vi "Main.vi"() -> ()   [LabVIEW 2020, in "Polar Bear Plus All-in-One Plugin.lvlib"]
doc: "Main user interface for the Polar Bear Plus Flow Synthesiser controller and plugin."
uses:
  Polar Bear Plus All-in-One Plugin.lvlib
  support/Message Queue/Message Queue.lvlib
  <vilib>/Utility/error.llb/Error Cluster From Error Code.vi
  <vilib>/ErrorRing/Error Ring.xnode
  support/User Event - Stop/User Event - Stop.lvlib
  process loops/UI Manager/UI Data.ctl
  Typedefs/System Control Data.ctl
  process loops/Acquisition/Acquisition.lvlib
  process loops/Instrument Manager/Instrument Manager.lvlib
  process loops/Remote Connection Manager/Remote Connection Manager.lvlib
  process loops/Logging/Logging.lvlib
  process loops/Instrument Manager/Instrument State.ctl
  process loops/UI Manager/UI Display State.ctl
  process loops/Logging/Logging Configuration.ctl
  process loops/UI Manager/Data Display Loop Data.ctl
  <instrlib>/RxnRover/Driver Polar Bear Plus/heater_parent/heater_parent.lvclass
panel:
  in  "Ramp Rate":dbl format="%.3f °C"
  out "Heat Switch Active":bool
  in  "Time Interval (sec)":i32=1200
  out "Temperature Graph":cluster{timestamp[], dbl[]}[](graph)
  in  "Config Log Btn":bool
  in  "Sampling rate\n(sec/sample)":dbl=1.0 min=0.1 step=0.1
  in  "Log Data":bool
  in  "Stop Btn":bool=TRUE
  in  "Run Btn":bool
  out "Temperature Ind":dbl format="%.3f °C"
  in  "Setpoint":dbl format="%.3f °C"
  # "Polar Bear Plus Heater"
  # "Config"
  # "Instrument Control"
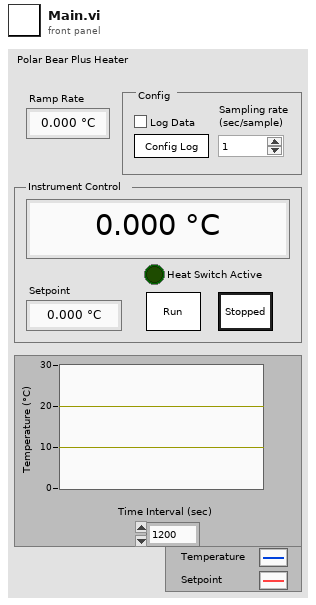
[diagram p1: front panel]
types:
  T1 = typedef "Polar Bear Plus All-in-One Plugin.lvlib/Data Display Loop Data.ctl" = cluster{"Data Timestamps":timestamp[], "Data Values":dbl[], "Setpoint":dbl[], "Previous Run State":bool}
  T2 = typedef "Polar Bear Plus All-in-One Plugin.lvlib/Instrument Manager.lvlib/Instrument State.ctl" = cluster{"Setpoint":dbl, "Running":bool, "Running Since":timestamp, "Data Point":cluster{"Time Stamp":timestamp, "Value":dbl}, "Sampling Rate (sec/sample)":dbl, "Ramp Rate":dbl, "Heat Switch Active?":bool, "Driver Object":refnum<class "heater_parent.lvclass">}
  T3 = typedef "Polar Bear Plus All-in-One Plugin.lvlib/Message Queue.lvlib/All Message Queues.ctl" = cluster{"System Control":refnum<queue>, "Instrument":refnum<queue>, "Remote":refnum<queue>, "UI":refnum<queue>, "Acquisition":refnum<queue>, "Logging":refnum<queue>}
  T4 = typedef "Polar Bear Plus All-in-One Plugin.lvlib/UI Display State.ctl" = enum16{"Shown", "Hidden"}
  T5 = enum8{"Enabled", "Disabled", "Disabled and Grayed Out"}
  T6 = typedef "Polar Bear Plus All-in-One Plugin.lvlib/UI Data.ctl" = cluster{"VISA Resource Ind":refnum<vi>, "Setpoint Ctl":refnum<vi>, "Run Btn":refnum<vi>, "Stop Btn":refnum<vi>, "Temperature Ind":refnum<vi>, "Log Data":refnum<vi>, "Config Log Btn":refnum<vi>, "Sampling rate\n(sec/sample)":refnum<vi>, "Temperature Graph":refnum<vi>}
  T7 = typedef "Polar Bear Plus All-in-One Plugin.lvlib/Logging.lvlib/Logging Configuration.ctl" = cluster{"Log Directory Path":path, "Log File Path":path, "Log File Prefix":string, "Log File Extension":string, "File Delimiter":string, "Header Info":string[][], "Channels":string[], "Log Instrument Runs":bool}
  T8 = typedef "Polar Bear Plus All-in-One Plugin.lvlib/System Control Data.ctl" = cluster{"Example Value <Replace Me>":dbl, "Log Runs":bool, "Clone":bool}
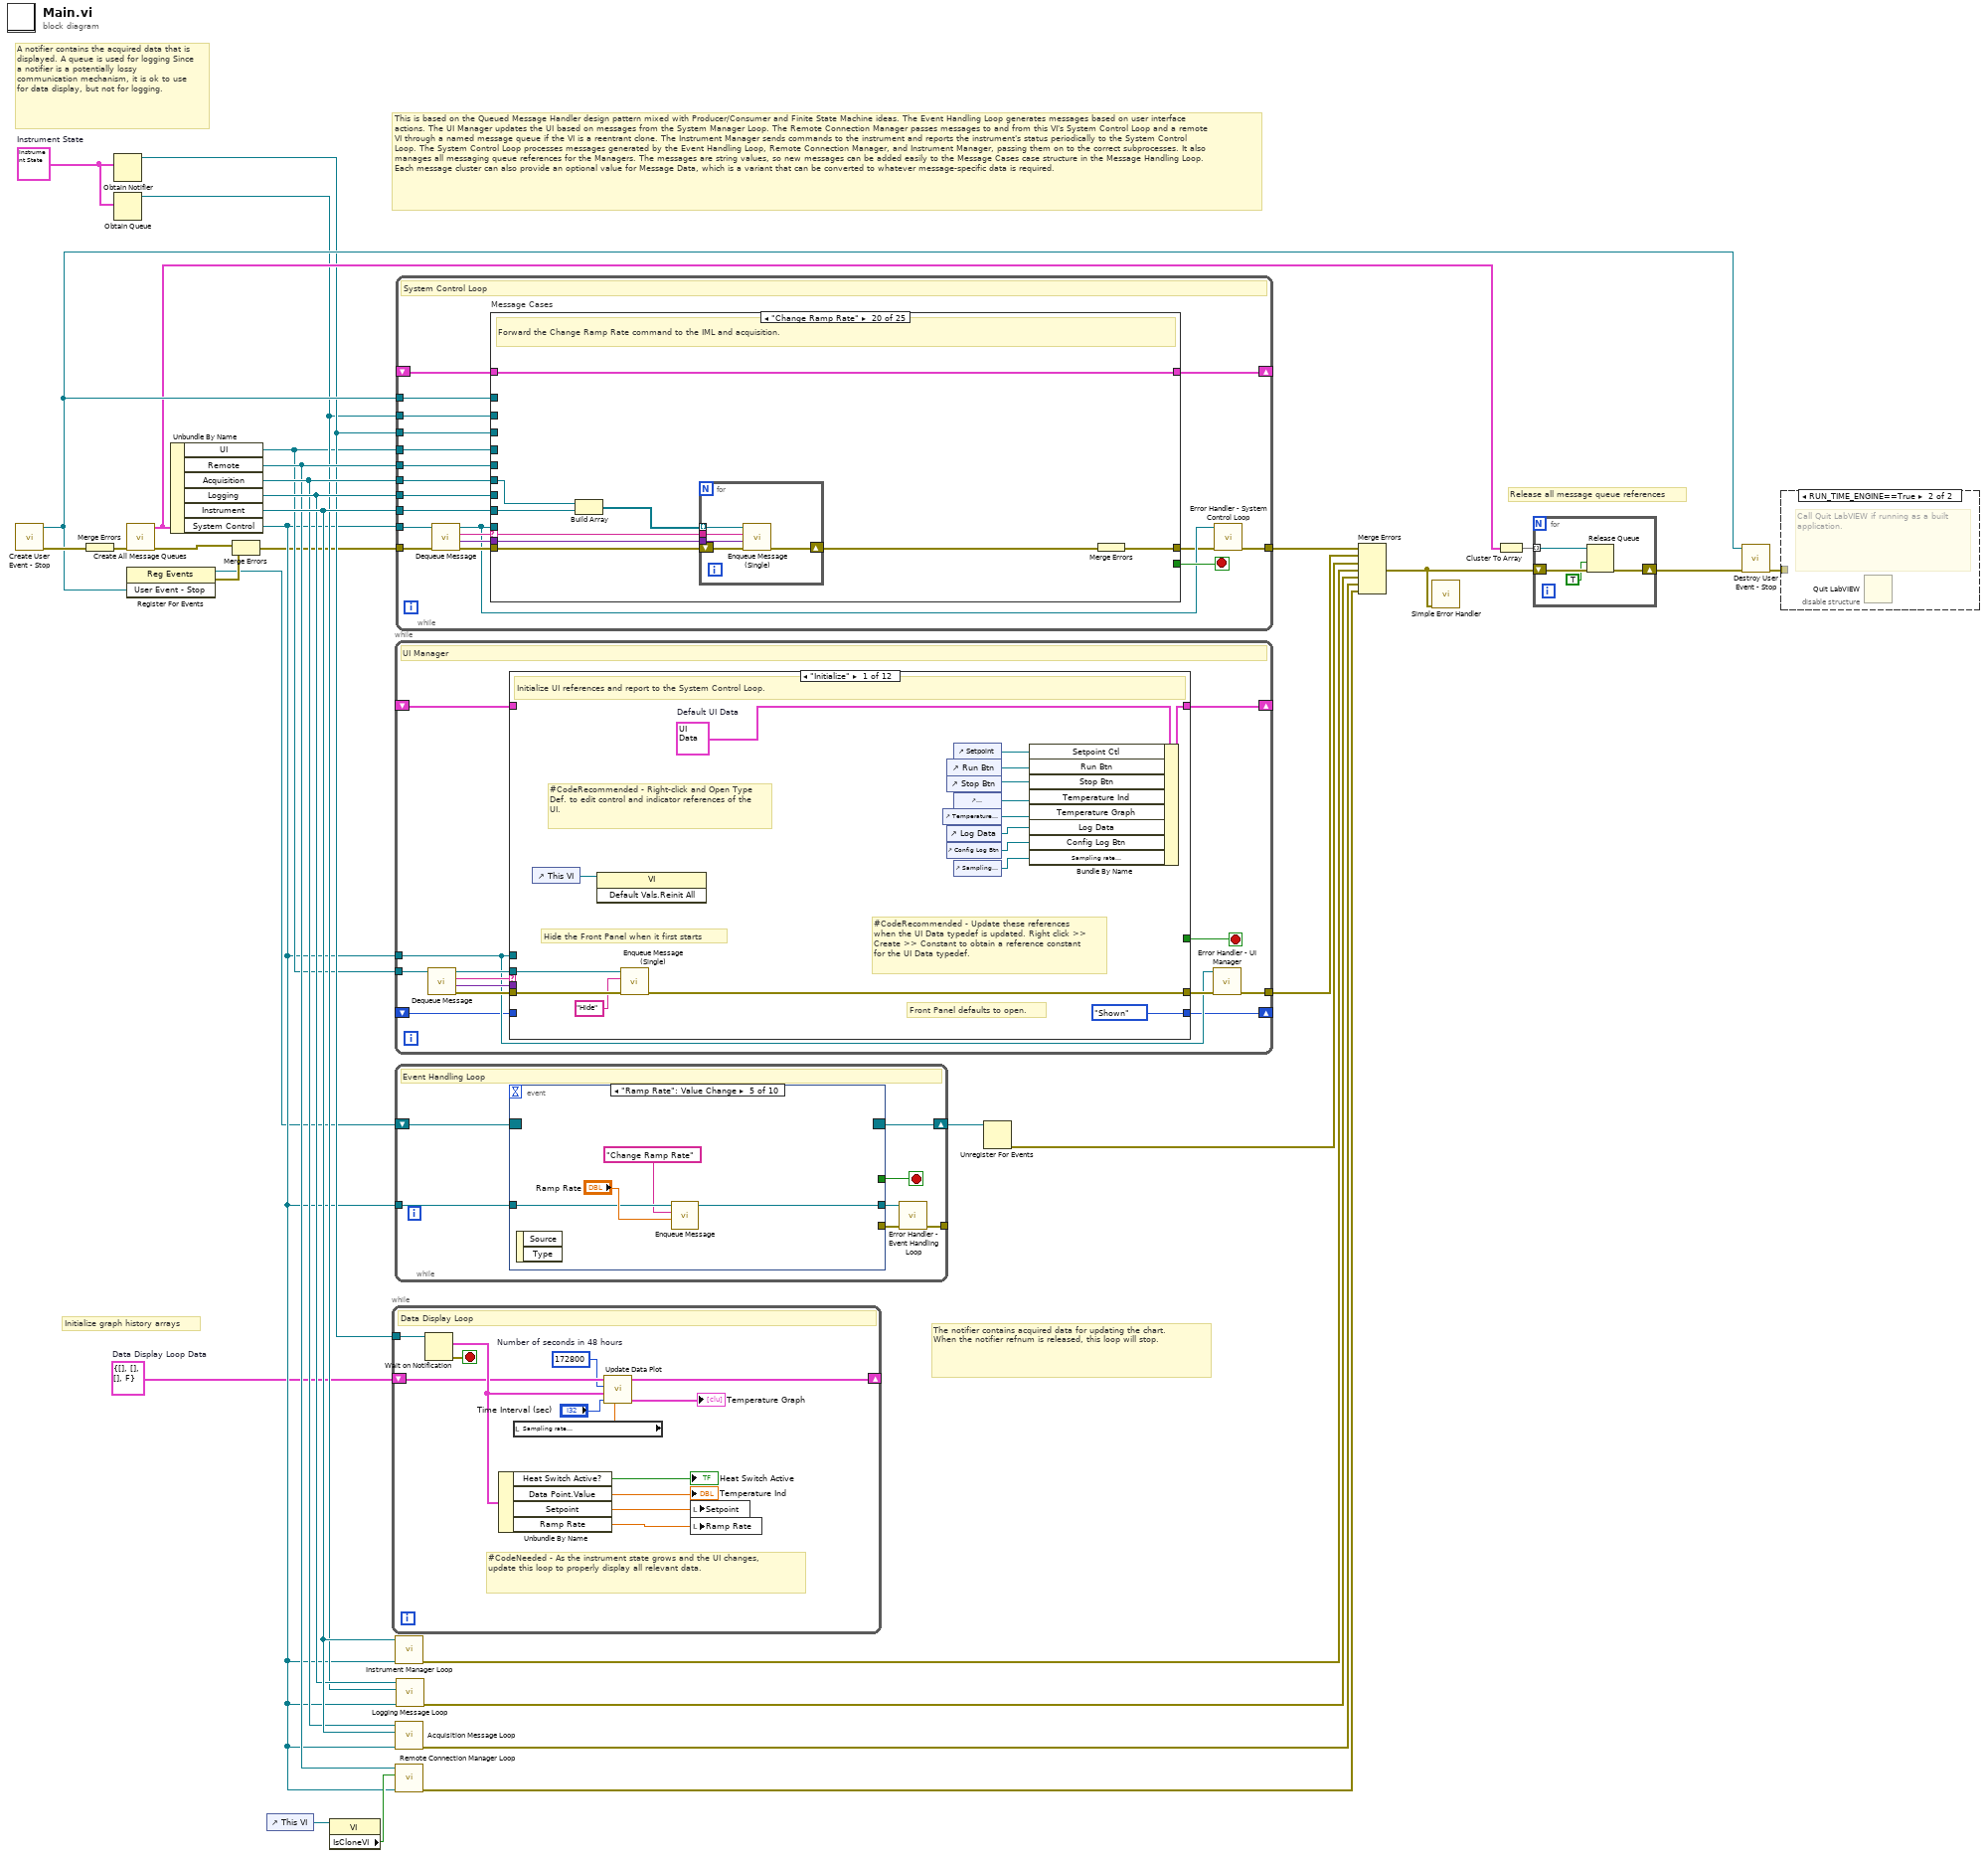
[diagram p0: block diagram]
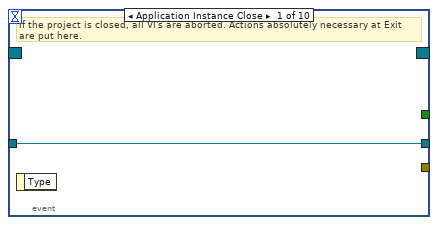
[diagram p2: hidden frame]
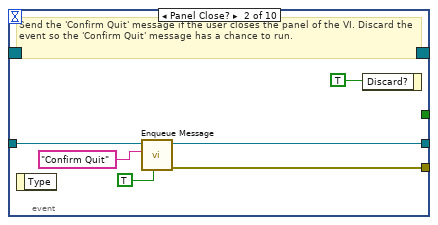
[diagram p3: hidden frame]
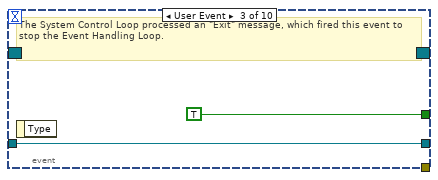
[diagram p4: hidden frame]
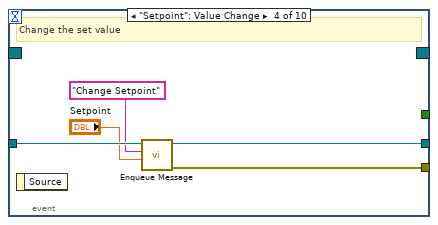
[diagram p5: hidden frame]
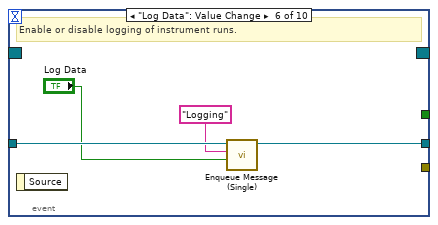
[diagram p6: hidden frame]
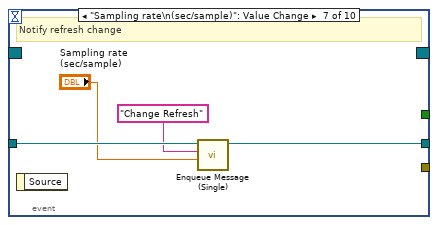
[diagram p7: hidden frame]
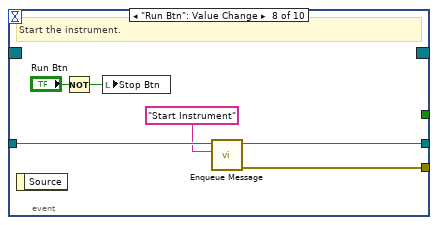
[diagram p8: hidden frame]
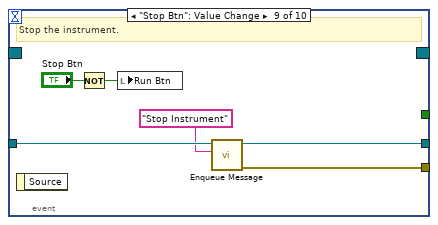
[diagram p9: hidden frame]
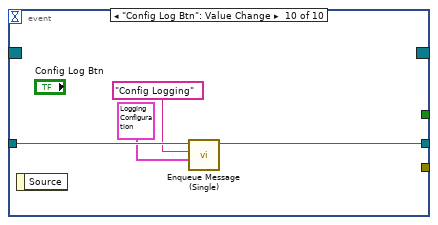
[diagram p10: hidden frame]
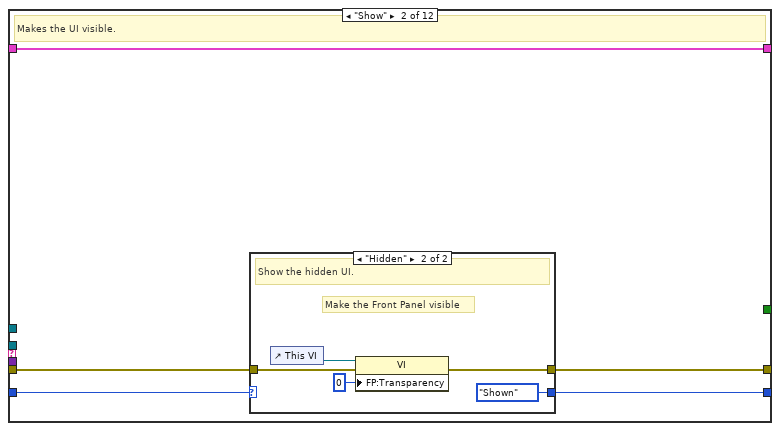
[diagram p11: hidden frame]
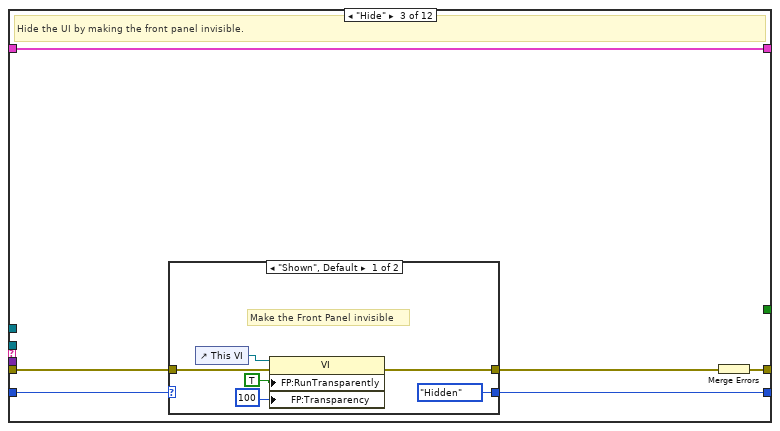
[diagram p13: hidden frame]
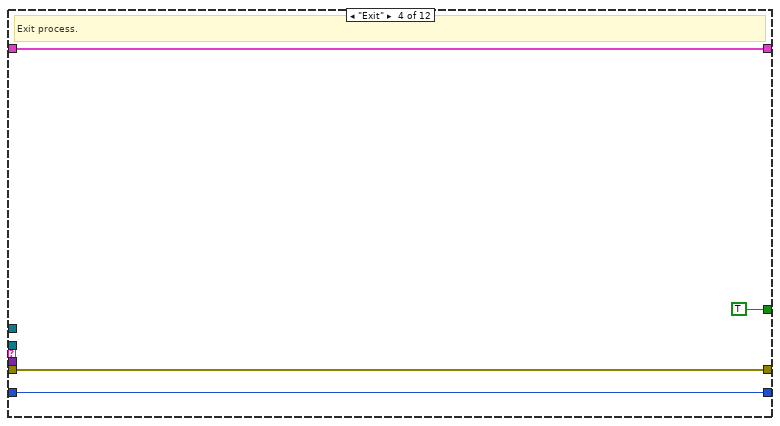
[diagram p15: hidden frame]
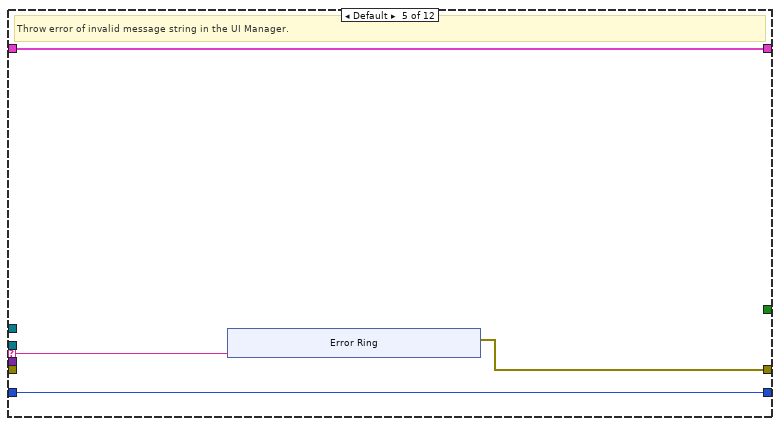
[diagram p16: hidden frame]
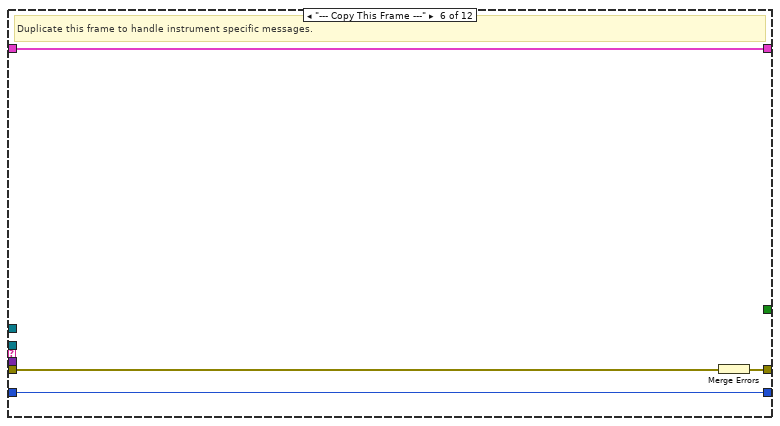
[diagram p17: hidden frame]
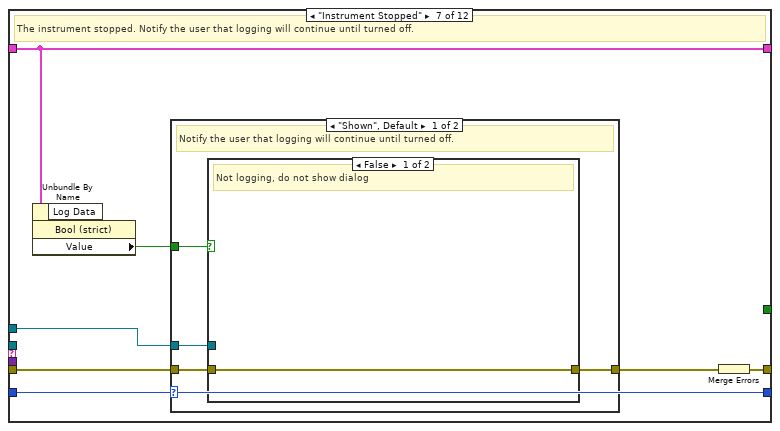
[diagram p18: hidden frame]
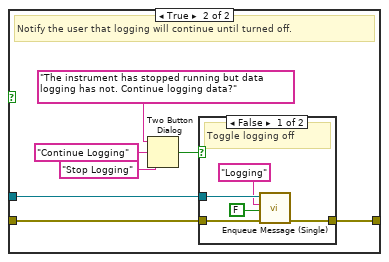
[diagram p19: hidden frame]
diagram:
  w1 = T1 {"Data Timestamps"=[], "Data Values"=[], "Setpoint"=[], "Previous Run State"=FALSE}  # Data Display Loop Data
  w7 = T2 {"Setpoint"=0.0, "Running"=FALSE, "Running Since"=timestamp(0 s since 1904-01-01), "Data Point"={"Time Stamp"=timestamp(0 s since 1904-01-01), "Value"=0.0}, "Sampling Rate (sec/sample)"=0.0, "Ramp Rate"=0.0, "Heat Switch Active?"=FALSE, "Driver Object"=refnum}  # Instrument State
  # "Initialize graph history arrays"
  # "A notifier contains the acquired data that is displayed. A queue is used for logging Since a notifier is a potentially lossy communication mechanism, it is ok to use for data display, but not for logging."
  # "The notifier contains acquired data for updating the chart. When the notifier refnum is released, this loop will stop."
  # "Release all message queue references"
  # "This is based on the Queued Message Handler design pattern mixed with Producer/Consumer and Finite State Machine ideas. The Event Handling Loop generates messages based on user interface actions. The UI Manager updates the UI based on messages from the System Manager Loop. The Remote Connection Manager passes messages to and from this VI's System Control Loop and a remote VI through a named message queue if the VI is a reentrant clone. The Instrument Manager sends commands to the instrument and reports the instrument's status periodically to the System Control Loop. The System Control Loop processes messages generated by the Event Handling Loop, Remote Connection Manager, and Instrument Manager, passing them on to the correct subprocesses. It also manages all messaging queue references for the Managers. The messages are string values, so new messages can be added easily to the Message Cases case structure in the Message Handling Loop.  Each message cluster can also provide an optional value for Message Data, which is a variant that can be converted to whatever message-specific data is required."
  n1 = call "Create User Event - Stop.vi"() -> ("error out"=w26:errorcluster, "User Event - Stop"=w22:refnum<user-event>)  [unwired: 10 in]
  n2 = Merge Errors(w26) -> (w25:errorcluster)
  n3 = Obtain Notifier(notification data type=w7) -> (notifier out=w8:refnum<notifier>)  [unwired: 3 in, 2 out]
  n4 = Obtain Queue(element data type=w7) -> (queue out=w6:refnum<queue>)  [unwired: 4 in, 2 out]
  n5 = call "Create All Message Queues.vi"("error in (no error)"=w25) -> ("error out"=w28:errorcluster, "Message Queues out"=w11:T3)  [unwired: 9 in]
  n6 = register-events(w22) -> (reference out=w2:refnum<event-registration>, error out=w13:errorcluster)  [unwired: 2 in]
  n7 = Unbundle By Name(w11) -> ("UI"=w5:refnum<queue>, "Remote"=w29:refnum<queue>, "Acquisition"=w30:refnum<queue>, "Logging"=w31:refnum<queue>, "Instrument"=w32:refnum<queue>, "System Control"=w4:refnum<queue>)
  n8 = Merge Errors(w28, w13) -> (w3:errorcluster)
  n9 = control-ref of="This VI"() -> (w21:refnum<vi>)
  n10 = property class="VI"(reference=w21) -> ("IsCloneVI"=w20:bool)  [unwired: 1 in, 2 out]
  n11 = while "Data Display Loop" {
    tunnel: w8 -> [w45]
    shift-right: [w38] -> _
    shift-left: w1 -> [w39]
    stop <- w44 stop-if-true
    w35 = 172800  # Number of seconds in 48 hours
    # "#CodeNeeded - As the instrument state grows and the UI changes, update this loop to properly display all relevant data."
    # "Data Display Loop"
    n12 = Wait on Notification(notifier=w45) -> (notification=w40:T2, error out=w44:errorcluster)  [unwired: 3 in, 2 out]
    n13 = Unbundle By Name(w40) -> ("Heat Switch Active?"=→"Heat Switch Active":bool, "Data Point.Value"=→"Temperature Ind":dbl, "Setpoint"=w42:dbl, "Ramp Rate"=w33:dbl)
    n14 = local read "Sampling rate\n(sec/sample)"() -> (w36:dbl)
    n15 = call "Update Data Plot.vi"("Sample Rate (sec/sample)"=w36, "Time interval (s)"="Time Interval (sec)", "Instrument State"=w40, "History length"=w35, "Graph History Arrays in"=w39) -> ("Updated Plot History"=→"Temperature Graph":cluster{timestamp[], dbl[]}[], "Graph History Arrays out"=w38:T1)  [unwired: 5 in]
    n16 = local write "Setpoint"(w42) -> ()
    n17 = local write "Ramp Rate"(w33) -> ()
  }
  n18 = while {
    tunnel: w5 -> [w58]
    tunnel: w4 -> [w49]
    tunnel: [w50] -> w19
    shift-right: [w53] -> _
    shift-left: _ -> [w52]
    shift-right: [w47] -> _
    shift-left: _ -> [w46]
    stop <- w48 stop-if-true
    # "UI Manager"
    n19 = call "Dequeue Message.vi"("Message Queue"=w58) -> ("error out"=w56:errorcluster, "Message Data"=w54:variant, "Message"=w55:string, "dup Message Queue"=w57:refnum<queue>)  [unwired: 7 in]
    n20 = case shown="\"Initialize\"" w55 {
      selector: w55 -> [_ _ _ _ w108 _ _ _ _ _ _ _]
      tunnel: w57 -> [w66 _ _ _ _ _ _ _ _ _ _ _]
      tunnel: w56 -> [w71 w78 w90 w104 _ w117 w125 w153 w161 w169 w180 w191]
      tunnel: w54 -> [_ _ _ _ _ _ _ _ _ w168 w178 w189]
      tunnel: w49 -> [_ _ _ _ _ _ w123 _ _ _ _ _]
      tunnel: [w67 w77 w91 w104 w107 w118 w127 w154 w162 w170 w181 w192] -> w51
      tunnel: [w73 w79 w92 w103 w106 w119 w122 w149 w155 w164 w172 w183] -> w53
      tunnel: w52 -> [_ w79 w92 w103 w106 w119 w122 w149 w155 w164 w172 w183]
      tunnel: [_ _ _ TRUE _ _ _ _ _ _ _ _] -> w48
      tunnel: w46 -> [_ w76 w88 w101 w105 w116 w126 w152 w160 w166 w173 w184]
      tunnel: [UI_Display_State."Shown" ("UI Display State") w75 w87 w101 w105 w116 w126 w152 w160 w166 w173 w184] -> w47
      frame "Initialize" {
        w74 = T6 {"VISA Resource Ind"=refnum, "Setpoint Ctl"=refnum, "Run Btn"=refnum, "Stop Btn"=refnum, "Temperature Ind"=refnum, "Log Data"=refnum, "Config Log Btn"=refnum, "Sampling rate\n(sec/sample)"=refnum, "Temperature Graph"=refnum}  # Default UI Data
        # "Front Panel defaults to open."
        # "Hide the Front Panel when it first starts"
        # "#CodeRecommended - Update these references when the UI Data typedef is updated. Right click >> Create >> Constant to obtain a reference constant for the UI Data typedef."
        # "#CodeRecommended - Right-click and Open Type Def. to edit control and indicator references of the UI."
        # "Initialize UI references and report to the System Control Loop."
        n21 = control-ref of="This VI"() -> (w59:refnum<vi>)
        n22 = invoke class="VI" method="Default Vals.Reinit All"(reference=w59) -> ()  [unwired: 2 in, 3 out]
        n23 = call "Enqueue Message (Single).vi"("error in (no error)"=w71, "Message"="Hide", "Message Queue"=w66) -> ("error out"=w67:errorcluster)  [unwired: 7 in, 1 out]
        n24 = control-ref of="Temperature Graph"() -> (w63:refnum<vi>)
        n25 = control-ref of="Run Btn"() -> (w69:refnum<vi>)
        n26 = control-ref of="Stop Btn"() -> (w70:refnum<vi>)
        n27 = control-ref of="Log Data"() -> (w62:refnum<vi>)
        n28 = control-ref of="Config Log Btn"() -> (w61:refnum<vi>)
        n29 = control-ref of="Setpoint"() -> (w72:refnum<vi>)
        n30 = control-ref of="Temperature Ind"() -> (w68:refnum<vi>)
        n31 = control-ref of="Sampling rate (sec/sample)"() -> (w60:refnum<vi>)
        n32 = Bundle By Name(cluster=w74, "Setpoint Ctl"=w72, "Run Btn"=w69, "Stop Btn"=w70, "Temperature Ind"=w68, "Temperature Graph"=w63, "Log Data"=w62, "Config Log Btn"=w61, "Sampling rate\n(sec/sample)"=w60) -> (w73:T6)
      }
      frame "Show" {
        # "Makes the UI visible."
        n33 = case shown="\"Hidden\"" w76 {
          selector: w76 -> [w81 _]
          tunnel: w78 -> [w80 w86]
          tunnel: [w80 w84] -> w77
          tunnel: [w81 UI_Display_State."Shown" ("UI Display State")] -> w75
          frame "Shown", Default {
            # "Do nothing if UI is already shown."
          }
          frame "Hidden" {
            # "Make the Front Panel visible"
            # "Show the hidden UI."
            n34 = control-ref of="This VI"() -> (w85:refnum<vi>)
            n35 = property class="VI"(reference=w85, error in=w86, "FP:Transparency"=u8 0 ("Front Panel Window:Transparency")) -> (error out=w84:errorcluster)  [unwired: 1 out]
          }
        }
      }
      frame "Hide" {
        # "Hide the UI by making the front panel invisible."
        n36 = case shown="\"Shown\", Default" w88 {
          selector: w88 -> [_ w100]
          tunnel: w90 -> [w95 w99]
          tunnel: [w94 w99] -> w89
          tunnel: [UI_Display_State."Hidden" ("UI Display State") w100] -> w87
          frame "Shown", Default {
            # "Make the Front Panel invisible"
            n37 = control-ref of="This VI"() -> (w98:refnum<vi>)
            n38 = property class="VI"(reference=w98, error in=w95, "FP:RunTransparently"=TRUE ("Front Panel Window:Run VI Transparently"), "FP:Transparency"=u8 100 ("Front Panel Window:Transparency")) -> (error out=w94:errorcluster)  [unwired: 1 out]
          }
          frame "Hidden" {
          }
        }
        n39 = Merge Errors(w89) -> (w91:errorcluster)
      }
      frame "Exit" {
        # "Exit process."
      }
      frame Default {
        # "Throw error of invalid message string in the UI Manager."
        n40 = xnode "Error Ring"("parameter 0"=w108) -> ("error out"=w107:errorcluster)
      }
      frame "--- Copy This Frame ---" {
        # "Duplicate this frame to handle instrument specific messages."
        n41 = Merge Errors(w117) -> (w118:errorcluster)
      }
      frame "Instrument Stopped" {
        # "The instrument stopped. Notify the user that logging will continue until turned off."
        n42 = Unbundle By Name(w122) -> ("Log Data"=w121:refnum<vi>)
        n43 = property class="Bool (strict)"(reference=w121) -> ("Value"=w120:bool)  [unwired: 1 in, 2 out]
        n44 = case shown="\"Shown\", Default" w126 {
          tunnel: w125 -> [w131 w146]
          tunnel: [w130 w146] -> w124
          tunnel: w123 -> [w129 _]
          tunnel: w120 -> [w128 _]
          frame "Shown", Default {
            # "Notify the user that logging will continue until turned off."
            n45 = case shown="False" w128 {
              tunnel: w131 -> [w132 w135]
              tunnel: [w132 w134] -> w130
              tunnel: w129 -> [_ w133]
              frame False {
                # "Not logging, do not show dialog"
              }
              frame True {
                # "Notify the user that logging will continue until turned off."
                n46 = Two Button Dialog(message="The instrument has stopped running but data logging has not. Continue logging data?", 1:"Stop Logging" ("F button name (\"Cancel\")"), 2:"Continue Logging" ("T button name (\"OK\")")) -> (T button?=w136:bool)
                n47 = case shown="False" w136 {
                  tunnel: w135 -> [w144 w145]
                  tunnel: [w143 w145] -> w134
                  tunnel: w133 -> [w142 _]
                  frame False {
                    # "Toggle logging off"
                    n48 = call "Enqueue Message (Single).vi"("error in (no error)"=w144, "Message Data"=FALSE, "Message"="Logging", "Message Queue"=w142) -> ("error out"=w143:errorcluster)  [unwired: 6 in, 1 out]
                  }
                  frame True {
                    # "Continues logging. Do nothing more"
                  }
                }
              }
            }
          }
          frame "Hidden" {
            # "Hidden, do not show dialog"
          }
        }
        n49 = Merge Errors(w124) -> (w127:errorcluster)
      }
      frame "Logging Started" {
        # "Indicate that logging started."
        n50 = Unbundle By Name(w149) -> ("Log Data"=w151:refnum<vi>)
        n51 = property class="Bool (strict)"(reference=w151, "Value"=TRUE ("Log Data")) -> ()  [unwired: 1 in, 2 out]
        n52 = Unbundle By Name(w149) -> ("Config Log Btn"=w148:refnum<vi>)
        n53 = property class="Bool"(reference=w148, "DisabledEnum"=T5."Disabled and Grayed Out" ("Disabled")) -> ()  [unwired: 1 in, 2 out]
        n54 = Merge Errors(w153) -> (w154:errorcluster)
      }
      frame "Logging Stopped" {
        # "Indicate that logging stopped."
        n55 = Unbundle By Name(w155) -> ("Log Data"=w159:refnum<vi>)
        n56 = property class="Bool (strict)"(reference=w159, "Value"=FALSE ("Log Data")) -> ()  [unwired: 1 in, 2 out]
        n57 = Unbundle By Name(w155) -> ("Config Log Btn"=w157:refnum<vi>)
        n58 = property class="Bool"(reference=w157, "DisabledEnum"=T5."Enabled" ("Disabled")) -> ()  [unwired: 1 in, 2 out]
        n59 = Merge Errors(w161) -> (w162:errorcluster)
      }
      frame "Change Refresh" {
        # "Update sample rate multiplier in the UI data chart and config indicator."
        n60 = Unbundle By Name(w164) -> ("Sampling rate\n(sec/sample)"=w165:refnum<vi>)
        n61 = Variant To Data(type=0.0, Variant=w168) -> (data=w163:dbl)  [unwired: 1 in, 1 out]
        n62 = property class="DigNum (strict)"(reference=w165, "Value"=w163) -> ()  [unwired: 1 in, 2 out]
        n63 = Merge Errors(w169) -> (w170:errorcluster)
      }
      frame "Display Units - Temperature Ind" {
        # "#CodeRecommended - If this format string is changed, update it on the front panel indicator as well."
        # "Change the units of the display."
        n64 = Variant To Data(type="", Variant=w178) -> (data=w176:string)  [unwired: 1 in, 1 out]
        n65 = call <vilib>:"Space Constant.vi"() -> ("String"=w177:string)
        n66 = Concatenate Strings("%.3f" ("string"), w177, w176) -> (w174:string)
        n67 = Unbundle By Name(w172) -> ("Temperature Ind"=w171:refnum<vi>)
        n68 = property on="Property Node" class="DigNum (strict)"(reference=w171, "FormatString"=w174) -> ()  [unwired: 1 in, 2 out]
        n69 = Merge Errors(w180) -> (w181:errorcluster)
      }
      frame "Display Units - Setpoint" {
        # "#CodeRecommended - If this format string is changed, update it on the front panel indicator as well."
        # "Change the units of the setpoint display."
        n70 = Variant To Data(type="", Variant=w189) -> (data=w187:string)  [unwired: 1 in, 1 out]
        n71 = call <vilib>:"Space Constant.vi"() -> ("String"=w188:string)
        n72 = Concatenate Strings("%.3f" ("string"), w188, w187) -> (w185:string)
        n73 = Unbundle By Name(w183) -> ("Setpoint Ctl"=w182:refnum<vi>)
        n74 = property on="Property Node" class="DigNum (strict)"(reference=w182, "FormatString"=w185) -> ()  [unwired: 1 in, 2 out]
        n75 = Merge Errors(w191) -> (w192:errorcluster)
      }
    }
    n76 = call "Error Handler - UI Manager.vi"("error in (no error)"=w51, "Message Queue"=w49) -> ("dup error in"=w50:errorcluster)  [unwired: 8 in, 1 out]
  }
  n77 = while {
    tunnel: w4 -> [w199]
    shift-right: [w197] -> w23
    shift-left: w2 -> [w198]
    tunnel: [w193] -> _
    stop <- w195 stop-if-true
    # "Event Handling Loop"
    n78 = event shown="[4] \"Ramp Rate\": Value Change" {
      selector: w198 -> [_ _ _ _ _ _ _ _ _ _]
      dyn-events: [_ _ _ _ _ _ _ _ _ _] -> w197
      timeout: _ -> [_ _ _ _ _ _ _ _ _ _]
      tunnel: [_ _ TRUE ("Discard?") _ _ _ _ _ _ _] -> w195
      tunnel: w199 -> [w200 w205 w208 w213 w216 w221 w225 w231 w237 w241]
      tunnel: [_ w204 _ w210 _ _ _ w229 w235 _] -> w196
      tunnel: [w200 w203 w208 w212 w215 w220 w224 w230 w236 w240] -> w194
      event Application Instance Close {
        # "If the project is closed, all VI's are aborted. Actions absolutely necessary at Exit are put here."
        n79 = event-data() -> ()  [unwired: 1 in, 1 out]
      }
      event Panel Close? {
        # "Send the 'Confirm Quit' message if the user closes the panel of the VI. Discard the event so the 'Confirm Quit' message has a chance to run."
        n80 = event-data() -> ()  [unwired: 1 in, 1 out]
        n81 = call-poly "Enqueue Message.vi"("Priority Message? (F)"=TRUE, "Message"="Confirm Quit", "Message Queue"=w205) -> ("error out"=w204:errorcluster, "dup Message Queue"=w203:refnum<queue>)  [unwired: 7 in]
        n82 = event-data("Discard?"=TRUE) -> ()  [unwired: 1 in, 1 out]
      }
      event User Event {
        # "The System Control Loop processed an \"Exit\" message, which fired this event to stop the Event Handling Loop."
        n83 = event-data() -> ()  [unwired: 1 in, 1 out]
      }
      event "Setpoint": Value Change {
        # "Change the set value"
        n84 = event-data() -> ()  [unwired: 1 in, 1 out]
        n85 = call-poly "Enqueue Message.vi"("Message Data"="Setpoint", "Message"="Change Setpoint", "Message Queue"=w213) -> ("error out"=w210:errorcluster, "dup Message Queue"=w212:refnum<queue>)  [unwired: 7 in]
      }
      event "Ramp Rate": Value Change {
        n86 = event-data() -> ()  [unwired: 1 in, 2 out]
        n87 = call-poly "Enqueue Message.vi"("Message Data"="Ramp Rate", "Message"="Change Ramp Rate", "Message Queue"=w216) -> ("dup Message Queue"=w215:refnum<queue>)  [unwired: 7 in, 1 out]
      }
      event "Log Data": Value Change {
        # "Enable or disable logging of instrument runs."
        n88 = event-data() -> ()  [unwired: 1 in, 1 out]
        n89 = call "Enqueue Message (Single).vi"("Message Data"="Log Data", "Message"="Logging", "Message Queue"=w221) -> ("dup Message Queue"=w220:refnum<queue>)  [unwired: 7 in, 1 out]
      }
      event "Sampling rate\n(sec/sample)": Value Change {
        # "Notify refresh change"
        n90 = event-data() -> ()  [unwired: 1 in, 1 out]
        n91 = call "Enqueue Message (Single).vi"("Message Data"="Sampling rate\n(sec/sample)", "Message"="Change Refresh", "Message Queue"=w225) -> ("dup Message Queue"=w224:refnum<queue>)  [unwired: 7 in, 1 out]
      }
      event "Run Btn": Value Change {
        # "Start the instrument."
        n92 = event-data() -> ()  [unwired: 1 in, 1 out]
        n93 = Not(x="Run Btn") -> (.not. x?=w226:bool)
        n94 = local write "Stop Btn"(w226) -> ()
        n95 = call-poly "Enqueue Message.vi"("Message"="Start Instrument", "Message Queue"=w231) -> ("error out"=w229:errorcluster, "dup Message Queue"=w230:refnum<queue>)  [unwired: 8 in]
      }
      event "Stop Btn": Value Change {
        # "Stop the instrument."
        n96 = event-data() -> ()  [unwired: 1 in, 1 out]
        n97 = Not(x="Stop Btn") -> (.not. x?=w232:bool)
        n98 = local write "Run Btn"(w232) -> ()
        n99 = call-poly "Enqueue Message.vi"("Message"="Stop Instrument", "Message Queue"=w237) -> ("error out"=w235:errorcluster, "dup Message Queue"=w236:refnum<queue>)  [unwired: 8 in]
      }
      event "Config Log Btn": Value Change {
        n100 = event-data() -> ()  [unwired: 1 in, 1 out]
        n101 = call "Enqueue Message (Single).vi"("Message Data"=T7 {"Log Directory Path"=path "", "Log File Path"=path "", "Log File Prefix"="Experiment", "Log File Extension"="csv", "File Delimiter"=",", "Header Info"=[], "Channels"=[], "Log Instrument Runs"=FALSE} ("Logging Configuration"), "Message"="Config Logging", "Message Queue"=w241) -> ("dup Message Queue"=w240:refnum<queue>)  [unwired: 7 in, 1 out]
      }
    }
    n102 = call "Error Handler - Event Handling Loop.vi"("error in (no error)"=w196, "Message Queue"=w194) -> ("dup error in"=w193:errorcluster)  [unwired: 8 in, 1 out]
  }
  n103 = call "Instrument Manager Loop.vi"("System Control"=w4, "Instrument Manager"=w32) -> ("error out"=w17:errorcluster)  [unwired: 9 in]
  n104 = call "Acquisition Message Loop.vi"("System Control"=w4, "Instrument Manager"=w32, "Acquisition"=w30) -> ("error out"=w15:errorcluster)  [unwired: 8 in]
  n105 = call "Remote Connection Manager Loop.vi"("System Control"=w4, "IsCloneVI (false)"=w20, "RCM Queue"=w29) -> ("error out"=w14:errorcluster)  [unwired: 8 in]
  n106 = while {
    tunnel: w4 -> [w252]
    shift-right: [w259] -> _
    shift-left: _ -> [w260]
    tunnel: w22 -> [w257]
    tunnel: w3 -> [w256]
    tunnel: [w250] -> w27
    tunnel: w32 -> [w248]
    tunnel: w29 -> [w247]
    tunnel: w5 -> [w246]
    tunnel: w30 -> [w245]
    tunnel: w31 -> [w244]
    tunnel: w8 -> [w243]
    tunnel: w6 -> [w242]
    stop <- w258 stop-if-true
    # "System Control Loop"
    n107 = call "Dequeue Message.vi"("error in (no error)"=w256, "Message Queue"=w252) -> ("error out"=w255:errorcluster, "Message Data"=w253:variant, "Message"=w254:string, "dup Message Queue"=w251:refnum<queue>)  [unwired: 6 in]
    n108 = case "Message Cases" shown="\"Change Ramp Rate\"" w254 {
      selector: w254 -> [_ _ _ w302 w315 w326 w344 w358 w364 _ w410 w417 w424 w431 w438 w448 w462 w477 w491 w505 w516 w523 w533 w548 w570]
      tunnel: w251 -> [_ _ w282 _ _ _ _ _ _ _ _ _ _ _ _ _ _ _ _ _ _ _ _ _ _]
      tunnel: w255 -> [w264 w279 w286 _ _ w329 w347 w362 w380 w393 w414 w421 w428 w435 w442 w451 w465 w481 w495 w509 w519 w526 _ _ _]
      tunnel: [w263 w273 w284 w305 w316 w335 w349 w363 w371 w398 w415 w422 w429 w436 w443 w452 w466 w479 w493 w507 w520 w527 w532 w547 w569] -> w249
      tunnel: w260 -> [_ w278 w285 w301 w317 w336 w350 w361 w370 w399 w416 w423 w430 w437 w444 w453 w467 w480 w494 w508 w521 w528 w531 w544 w567]
      tunnel: [w265 w278 w285 w301 w317 w336 w350 w361 w370 w397 w416 w423 w430 w437 w444 w453 w467 w480 w494 w508 w521 w528 w531 w544 w567] -> w259
      tunnel: [_ _ _ TRUE _ _ _ _ _ _ _ _ _ _ _ _ _ _ _ _ _ _ _ _ _] -> w258
      tunnel: w253 -> [_ w277 _ w306 _ w325 w343 w357 w365 w395 w411 w418 w425 w432 w439 w449 w463 w476 w490 w504 w517 w524 w534 w549 w565]
      tunnel: w257 -> [_ _ _ w303 _ _ _ _ _ _ _ _ _ _ _ _ _ _ _ _ _ _ _ _ _]
      tunnel: w248 -> [w262 _ _ w298 _ w330 _ w359 _ _ _ _ _ _ _ _ _ _ w489 w503 w515 w522 _ _ _]
      tunnel: w247 -> [_ _ _ w297 _ w333 w348 _ w375 _ _ _ _ _ _ w447 w461 _ _ _ _ _ w535 w545 w568]
      tunnel: w246 -> [_ _ _ w296 _ w332 _ _ w374 _ _ _ _ _ _ w446 w460 w474 _ _ _ _ _ w543 _]
      tunnel: w245 -> [_ _ _ w300 _ w334 _ _ w377 _ _ _ _ _ _ _ _ w475 w488 w502 _ _ w530 _ _]
      tunnel: w244 -> [_ _ _ w299 _ w331 _ _ w367 w391 w412 w419 w426 w433 w440 _ _ _ _ _ _ _ w529 _ _]
      tunnel: w243 -> [_ _ _ w293 _ _ _ _ _ _ _ _ _ _ _ _ _ _ _ _ _ _ _ _ w566]
      tunnel: w242 -> [_ _ _ w291 _ _ _ _ _ _ _ _ _ _ _ _ _ _ _ _ _ _ _ _ w562]
      frame "Initialize" {
        w266 = T8 {"Example Value <Replace Me>"=0.0, "Log Runs"=FALSE, "Clone"=FALSE}  # Default Data
        # "Initialize the system control loop and system."
        n109 = control-ref of="This VI"() -> ()  [unwired: 1 out]
        n110 = property on="Property Node" class="VI"() -> ("IsCloneVI"=w261:bool)  [unwired: 2 in, 2 out]
        n111 = Bundle By Name(cluster=w266, "Clone"=w261) -> (w265:T8)
        n112 = case shown="False" w261 {
          tunnel: w264 -> [w269 w272]
          tunnel: [w268 w272] -> w263
          tunnel: w262 -> [w267 _]
          frame False {
            # "Initiate the VISA Resource selection window if this is not a"
            n113 = call "Enqueue Message (Single).vi"("error in (no error)"=w269, "Message Data"=refnum<visa-resource-name> refnum ("VISA resource out"), "Message"="Set VISA Resource", "Message Queue"=w267) -> ("error out"=w268:errorcluster)  [unwired: 6 in, 1 out]
          }
          frame True {
            # "Reentrant clone. It is the responsibility of the RCM to send the Set VISA Resource command."
          }
        }
      }
      frame "Error" {
        # "#CodeRecommended - If you ever change the name of this \"Error\" message, you'll need to update the name in the Check Loop Error.vi as well."
        # "#CodeRecommended - Consider creating a system for logging errors in some way. These errors are for notification purposes only. Handling of specific errors should be performed in the message frames that generated the error."
        # "Error - Display an error dialog. This message is sent by the \"Error Handler\" VIs at the end of other loops in this application."
        n114 = Variant To Data(error in=w279, type=errorcluster {"status"=FALSE, "code"=0, "source"=""} ("error constant"), Variant=w277) -> (data=w275:errorcluster, error out=w274:errorcluster)
        n115 = call <vilib>:"Simple Error Handler.vi"("error in (no error)"=w275) -> ()  [unwired: 4 in, 5 out]
        n116 = Merge Errors(w274) -> (w273:errorcluster)
      }
      frame "Confirm Quit" {
        # "#CodeNeeded - If you want to provide an \"Are you sure\" dialog (or some other notification) before the application exits, place that code here. This message is typically sent from a Panel Close? event."
        # "Confirm Quit - Message that can confirm whether or not the user wants to exit the application."
        n117 = call-poly "Enqueue Message.vi"("Priority Message? (F)"=TRUE, "error in (no error)"=w286, "Message"="Exit", "Message Queue"=w282) -> ("error out"=w283:errorcluster)  [unwired: 6 in, 1 out]
        n118 = Merge Errors(w283) -> (w284:errorcluster)
      }
      frame "Exit" {
        # "Order other processes to exit"
        # "Begin the application closing procedure by sending \"Exit\" commands to all running processes."
        n119 = Variant To Data(type=errorcluster {"status"=FALSE, "code"=0, "source"=""} ("error constant"), Variant=w306) -> (data=w307:errorcluster)  [unwired: 1 in, 1 out]
        n120 = Build Array(w296, w297, w300, w299, w298) -> (w295:refnum<queue>[])
        n121 = call <vilib>:"Clear Errors.vi"("error in (no error)"=w307, "specific error code to clear (0: all)"=5000) -> ("error out"=w288:errorcluster)  [unwired: 4 in, 1 out]
        n122 = call <vilib>:"Simple Error Handler.vi"("error in (no error)"=w288) -> ()  [unwired: 4 in, 5 out]
        n123 = for {
          tunnel: w302 -> [w313]
          tunnel: w295 -> [w312] mode=indexing
          shift-right: [w311] -> w304
          shift-left: _ -> [w310]
          n124 = call "Enqueue Message (Single).vi"("Priority Message? (F)"=TRUE, "Message"=w313, "Message Queue"=w312) -> ("error out"=w314:errorcluster)  [unwired: 7 in, 1 out]
          n125 = Merge Errors(w314, w310) -> (w311:errorcluster)
        }
        n126 = Release Notifier(notifier=w293) -> (error out=w292:errorcluster)  [unwired: 2 in, 2 out]
        n127 = Release Queue(queue=w291) -> (error out=w289:errorcluster)  [unwired: 2 in, 2 out]
        n128 = call "Fire User Event - Stop.vi"("User Event - Stop"=w303) -> ("error out"=w290:errorcluster)  [unwired: 10 in]
        n129 = Merge Errors(w290, w289, w292, w304) -> (w305:errorcluster)
      }
      frame Default {
        # "'Default' case only runs if there is a message that isn't defined in any of the other cases.  Output a programming error."
        n130 = xnode "Error Ring"("parameter 0"=w315) -> ("error out"=w316:errorcluster)
      }
      frame "---Copy This Frame---" {
        # "Sends the message to each process in the array."
        # "#CodeRecommended - Change connections to build an array of the processes that will receive this message"
        # "Duplicate this frame when creating new messages.  Change this comment in the duplicated frame to describe this message."
        n131 = Build Array(w332, w333, w334, w331, w330) -> (w327:refnum<queue>[])
        n132 = for {
          tunnel: w327 -> [w340] mode=indexing
          tunnel: w326 -> [w342]
          tunnel: w325 -> [w341]
          shift-right: [w339] -> w328
          shift-left: w329 -> [w337]
          n133 = call "Enqueue Message (Single).vi"("Message Data"=w341, "Message"=w342, "Message Queue"=w340) -> ("error out"=w338:errorcluster)  [unwired: 7 in, 1 out]
          n134 = Merge Errors(w338, w337) -> (w339:errorcluster)
        }
        n135 = Merge Errors(w328) -> (w335:errorcluster)
      }
      frame "Set Remote Queue" {
        # "Sends the message to each process in the array."
        # "Bounce this message back to the Remote Control Manager to set the remote queue to publish messages to."
        n136 = Build Array(w348) -> (w345:refnum<queue>[])
        n137 = for {
          tunnel: w345 -> [w354] mode=indexing
          tunnel: w344 -> [w356]
          tunnel: w343 -> [w355]
          shift-right: [w353] -> w346
          shift-left: w347 -> [w351]
          n138 = call "Enqueue Message (Single).vi"("Message Data"=w355, "Message"=w356, "Message Queue"=w354) -> ("error out"=w352:errorcluster)  [unwired: 7 in, 1 out]
          n139 = Merge Errors(w352, w351) -> (w353:errorcluster)
        }
        n140 = Merge Errors(w346) -> (w349:errorcluster)
      }
      frame "Set VISA Resource" {
        # "Update the VISA Resource of the instrument."
        n141 = call "Enqueue Message (Single).vi"("error in (no error)"=w362, "Message Data"=w357, "Message"=w358, "Message Queue"=w359) -> ("error out"=w360:errorcluster)  [unwired: 6 in, 1 out]
        n142 = Merge Errors(w360) -> (w363:errorcluster)
      }
      frame "Valid VISA Resource" {
        # "When a Valid VISA Resource has been chosen, start the other processes."
        n143 = Unbundle By Name(w370) -> ("Log Runs"=w369:bool)
        n144 = call "Enqueue Message (Single).vi"("error in (no error)"=w380, "Message Data"=w365, "Message"=w364, "Message Queue"=w367) -> ("error out"=w368:errorcluster, "dup Message Queue"=w366:refnum<queue>)  [unwired: 6 in]
        n145 = case shown="True" w369 {
          tunnel: w368 -> [w381 w385]
          tunnel: w366 -> [_ w384]
          tunnel: [w381 w382] -> w378
          frame False {
          }
          frame True {
            n146 = call "Enqueue Message (Single).vi"("error in (no error)"=w385, "Message"="Start", "Message Queue"=w384) -> ("error out"=w382:errorcluster)  [unwired: 7 in, 1 out]
          }
        }
        n147 = call "Enqueue Message (Single).vi"("error in (no error)"=w378, "Message"="Start", "Message Queue"=w377) -> ("error out"=w376:errorcluster)  [unwired: 7 in, 1 out]
        n148 = Unbundle By Name(w370) -> ("Clone"=w372:bool)
        n149 = call "Enqueue Message (Single).vi"("error in (no error)"=w376, "Message Data"=w365, "Message"=w364, "Message Queue"=w375) -> ("error out"=w373:errorcluster)  [unwired: 6 in, 1 out]
        n150 = case shown="False" w372 {
          tunnel: w373 -> [w389 w390]
          tunnel: [w388 w390] -> w371
          tunnel: w374 -> [w387 _]
          frame False {
            # "Show the Front Panel automatically on startup"
            n151 = call "Enqueue Message (Single).vi"("error in (no error)"=w389, "Message"="Show", "Message Queue"=w387) -> ("error out"=w388:errorcluster)  [unwired: 7 in, 1 out]
          }
          frame True {
            # "Reentrant clone. It is the responsibility of the RCM to send \"Show\"."
          }
        }
      }
      frame "Logging" {
        # "Enable or disable logging in the System Data. Run logging is disabled by default."
        n152 = Variant To Data(type=TRUE, Variant=w395) -> (data=w394:bool)  [unwired: 1 in, 1 out]
        n153 = case shown="True" w394 {
          tunnel: w393 -> [w404 w409]
          tunnel: [w403 w408] -> w392
          tunnel: w391 -> [w402 w407]
          frame False {
            n154 = call "Enqueue Message (Single).vi"("Priority Message? (F)"=TRUE, "error in (no error)"=w404, "Message"="Stop", "Message Queue"=w402) -> ("error out"=w403:errorcluster)  [unwired: 6 in, 1 out]
          }
          frame True {
            n155 = call "Enqueue Message (Single).vi"("Priority Message? (F)"=TRUE, "error in (no error)"=w409, "Message"="Start", "Message Queue"=w407) -> ("error out"=w408:errorcluster)  [unwired: 6 in, 1 out]
          }
        }
        n156 = Bundle By Name(cluster=w399, "Log Runs"=w394) -> (w397:T8)
        n157 = Merge Errors(w392) -> (w398:errorcluster)
      }
      frame "Config Logging" {
        # "Pass on Config Logging message to Logging Loop."
        n158 = call "Enqueue Message (Single).vi"("error in (no error)"=w414, "Message Data"=w411, "Message"=w410, "Message Queue"=w412) -> ("error out"=w413:errorcluster)  [unwired: 6 in, 1 out]
        n159 = Merge Errors(w413) -> (w415:errorcluster)
      }
      frame "Set Log Directory" {
        # "Pass on log setting message to Logging Loop."
        n160 = call "Enqueue Message (Single).vi"("error in (no error)"=w421, "Message Data"=w418, "Message"=w417, "Message Queue"=w419) -> ("error out"=w420:errorcluster)  [unwired: 6 in, 1 out]
        n161 = Merge Errors(w420) -> (w422:errorcluster)
      }
      frame "Set Log File Prefix" {
        # "Pass on log setting message to Logging Loop."
        n162 = call "Enqueue Message (Single).vi"("error in (no error)"=w428, "Message Data"=w425, "Message"=w424, "Message Queue"=w426) -> ("error out"=w427:errorcluster)  [unwired: 6 in, 1 out]
        n163 = Merge Errors(w427) -> (w429:errorcluster)
      }
      frame "Set Log File Delimiter" {
        # "Pass on log setting message to Logging Loop."
        n164 = call "Enqueue Message (Single).vi"("error in (no error)"=w435, "Message Data"=w432, "Message"=w431, "Message Queue"=w433) -> ("error out"=w434:errorcluster)  [unwired: 6 in, 1 out]
        n165 = Merge Errors(w434) -> (w436:errorcluster)
      }
      frame "Set Log on Run" {
        # "Pass on log setting message to Logging Loop."
        n166 = call "Enqueue Message (Single).vi"("error in (no error)"=w442, "Message Data"=w439, "Message"=w438, "Message Queue"=w440) -> ("error out"=w441:errorcluster)  [unwired: 6 in, 1 out]
        n167 = Merge Errors(w441) -> (w443:errorcluster)
      }
      frame "Logging Started" {
        # "Pass on Logging Started message to RCM and UI."
        n168 = Build Array(w446, w447) -> (w445:refnum<queue>[])
        n169 = for {
          tunnel: w449 -> [w456]
          tunnel: w448 -> [w455]
          shift-right: [w457] -> w450
          shift-left: w451 -> [w458]
          tunnel: w445 -> [w454] mode=indexing
          n170 = call "Enqueue Message (Single).vi"("error in (no error)"=w458, "Message Data"=w456, "Message"=w455, "Message Queue"=w454) -> ("error out"=w457:errorcluster)  [unwired: 6 in, 1 out]
        }
        n171 = Merge Errors(w450) -> (w452:errorcluster)
      }
      frame "Logging Stopped" {
        # "Pass on Logging Stopped message to RCM and UI."
        n172 = Build Array(w460, w461) -> (w459:refnum<queue>[])
        n173 = for {
          tunnel: w463 -> [w470]
          tunnel: w462 -> [w469]
          shift-right: [w471] -> w464
          shift-left: w465 -> [w472]
          tunnel: w459 -> [w468] mode=indexing
          n174 = call "Enqueue Message (Single).vi"("error in (no error)"=w472, "Message Data"=w470, "Message"=w469, "Message Queue"=w468) -> ("error out"=w471:errorcluster)  [unwired: 6 in, 1 out]
        }
        n175 = Merge Errors(w464) -> (w466:errorcluster)
      }
      frame "Change Refresh" {
        # "#CodeRecommended - If the default refresh time is changed, it must be updated in the UI and Data Acquisition Loop Data typedef."
        # "Change the sampling rate of the instrument. Default is 1 second/sample."
        n176 = Build Array(w474, w475) -> (w473:refnum<queue>[])
        n177 = for {
          tunnel: w477 -> [w484]
          tunnel: w476 -> [w483]
          tunnel: w473 -> [w482] mode=indexing
          shift-right: [w485] -> w478
          shift-left: w481 -> [w486]
          n178 = call "Enqueue Message (Single).vi"("error in (no error)"=w486, "Message Data"=w483, "Message"=w484, "Message Queue"=w482) -> ("error out"=w485:errorcluster)  [unwired: 6 in, 1 out]
        }
        n179 = Merge Errors(w478) -> (w479:errorcluster)
      }
      frame "Change Setpoint" {
        # "Forward the Change Setpoint command to the IML and acquisition."
        n180 = Build Array(w488, w489) -> (w487:refnum<queue>[])
        n181 = for {
          tunnel: w491 -> [w498]
          tunnel: w490 -> [w497]
          shift-right: [w499] -> w492
          shift-left: w495 -> [w500]
          tunnel: w487 -> [w496] mode=indexing
          n182 = call "Enqueue Message (Single).vi"("error in (no error)"=w500, "Message Data"=w497, "Message"=w498, "Message Queue"=w496) -> ("error out"=w499:errorcluster)  [unwired: 6 in, 1 out]
        }
        n183 = Merge Errors(w492) -> (w493:errorcluster)
      }
      frame "Change Ramp Rate" {
        # "Forward the Change Ramp Rate command to the IML and acquisition."
        n184 = Build Array(w502, w503) -> (w501:refnum<queue>[])
        n185 = for {
          tunnel: w505 -> [w512]
          tunnel: w504 -> [w511]
          shift-right: [w513] -> w506
          shift-left: w509 -> [w514]
          tunnel: w501 -> [w510] mode=indexing
          n186 = call "Enqueue Message (Single).vi"("error in (no error)"=w514, "Message Data"=w511, "Message"=w512, "Message Queue"=w510) -> ("error out"=w513:errorcluster)  [unwired: 6 in, 1 out]
        }
        n187 = Merge Errors(w506) -> (w507:errorcluster)
      }
      frame "Start Instrument" {
        # "Pass message to Instrument Manager Loop."
        n188 = call "Enqueue Message (Single).vi"("error in (no error)"=w519, "Message Data"=w517, "Message"=w516, "Message Queue"=w515) -> ("error out"=w518:errorcluster)  [unwired: 6 in, 1 out]
        n189 = Merge Errors(w518) -> (w520:errorcluster)
      }
      frame "Stop Instrument" {
        # "Pass message to Instrument Manager Loop."
        n190 = call "Enqueue Message (Single).vi"("error in (no error)"=w526, "Message Data"=w524, "Message"=w523, "Message Queue"=w522) -> ("error out"=w525:errorcluster)  [unwired: 6 in, 1 out]
        n191 = Merge Errors(w525) -> (w527:errorcluster)
      }
      frame "Instrument Started" {
        # "Build an array of all processes that will receive this message"
        # "Notify processes of update"
        # "Notify processes that the instrument is running."
        n192 = Build Array(w535, w530, w529) -> (w536:refnum<queue>[])
        n193 = for {
          tunnel: w536 -> [w540] mode=indexing
          tunnel: w533 -> [w542]
          tunnel: w534 -> [w541]
          shift-right: [w539] -> w532
          shift-left: _ -> [w537]
          n194 = call "Enqueue Message (Single).vi"("Message Data"=w541, "Message"=w542, "Message Queue"=w540) -> ("error out"=w538:errorcluster)  [unwired: 7 in, 1 out]
          n195 = Merge Errors(w538, w537) -> (w539:errorcluster)
        }
      }
      frame "Instrument Stopped" {
        # "Build an array of all processes that will receive this message"
        # "Notify processes of update"
        # "Notify processes that the instrument stopped running."
        n196 = Build Array(w543, w545) -> (w546:refnum<queue>[])
        n197 = for {
          tunnel: w546 -> [w553] mode=indexing
          tunnel: w548 -> [w555]
          tunnel: w549 -> [w554]
          shift-right: [w552] -> w547
          shift-left: _ -> [w550]
          n198 = call "Enqueue Message (Single).vi"("Message Data"=w554, "Message"=w555, "Message Queue"=w553) -> ("error out"=w551:errorcluster)  [unwired: 7 in, 1 out]
          n199 = Merge Errors(w551, w550) -> (w552:errorcluster)
        }
      }
      frame "Report" {
        # "Send instrument state notification"
        # "Notify processes that the instrument stopped running."
        n200 = Variant To Data(type=T2 {"Setpoint"=0.0, "Running"=FALSE, "Running Since"=timestamp(0 s since 1904-01-01), "Data Point"={"Time Stamp"=timestamp(0 s since 1904-01-01), "Value"=0.0}, "Sampling Rate (sec/sample)"=0.0, "Ramp Rate"=0.0, "Heat Switch Active?"=FALSE, "Driver Object"=refnum} ("Instrument State"), Variant=w565) -> (data=w561:T2)  [unwired: 1 in, 1 out]
        n201 = local read "Sampling rate\n(sec/sample)"() -> (w556:dbl)
        n202 = Bundle By Name(cluster=w561, "Sampling Rate (sec/sample)"=w556) -> (w557:T2)
        n203 = Enqueue Element(queue=w562, element=w557) -> (error out=w559:errorcluster)  [unwired: 2 in, 2 out]
        n204 = Send Notification(notification=w557, notifier=w566) -> (error out=w563:errorcluster)  [unwired: 1 in, 1 out]
        n205 = Merge Errors(w559, w563) -> (w560:errorcluster)
        n206 = call "Enqueue Message (Single).vi"("Message Data"=w557, "Message"=w570, "Message Queue"=w568) -> ("error out"=w558:errorcluster)  [unwired: 7 in, 1 out]
        n207 = Merge Errors(w558, w560) -> (w569:errorcluster)
      }
    }
    n208 = call "Error Handler - System Control Loop.vi"("error in (no error)"=w249, "Message Queue"=w251) -> ("dup error in"=w250:errorcluster)  [unwired: 8 in, 1 out]
  }
  n209 = call "Logging Message Loop.vi"("System Control"=w4, "Data Queue"=w6, "Logging"=w31) -> ("error out"=w16:errorcluster)  [unwired: 8 in]
  n210 = Unregister For Events(event registration refnum=w23) -> (error out=w18:errorcluster)  [unwired: 1 in]
  n211 = Merge Errors(w27, w19, w18, w17, w16, w15, w14) -> (w12:errorcluster)
  n212 = call <vilib>:"Simple Error Handler.vi"("error in (no error)"=w12) -> ()  [unwired: 4 in, 5 out]
  n213 = Cluster To Array(cluster=w11) -> (array=w10:refnum<queue>[])
  n214 = for {
    shift-right: [w572] -> w9
    shift-left: w12 -> [w573]
    tunnel: w10 -> [w574] mode=indexing
    n215 = Release Queue(queue=w574, force destroy? (F)=TRUE, error in (no error)=w573) -> (error out=w572:errorcluster)  [unwired: 2 out]
  }
  n216 = call "Destroy User Event - Stop.vi"("error in (no error)"=w9, "User Event - Stop"=w22) -> ("error out"=w24:errorcluster)  [unwired: 9 in]
  n217 = disable-structure shown="RUN_TIME_ENGINE==True" {
    disable-tunnel: w24 -> [_ _]
    frame condition #0 (active) {
    }
    frame condition #1 {
      # "Call Quit LabVIEW if running as a built application."
      n218 = Quit LabVIEW() -> ()  [unwired: 1 in]
    }
  }
